vi "XYZ stage control.vi"() -> ()   [LabVIEW 2020]
panel:
  in  "Z down step size":dbl=100.0
  in  "Y down step size":dbl=100.0
  in  "X down step size":dbl=100.0
  out "X Position":dbl=-10.99177734375
  in  "X Step Size(um)":dbl=100.0
  in  "Right":bool
  in  "Left":bool
  out "Y Position":dbl=3.8870703125000023
  in  "Focus Down X":bool
  in  "Y Step Size(um)":dbl=100.0
  in  "Focus Up X":bool caption="Focus Up"
  in  "Focus Down":bool
  out "Z Position":dbl=6.860690000000502
  in  "Focus Up":bool
  in  "Z step size (um)":dbl=100.0
  in  "Close Communication":bool
  out "Error out":errorcluster
  out "Connected":bool=TRUE
  out "GetFirmwareVersion 2":string="3.03\r"
  in  "SPIIPLUSCOM660Lib.IAsyncChannel":refnum<k7>
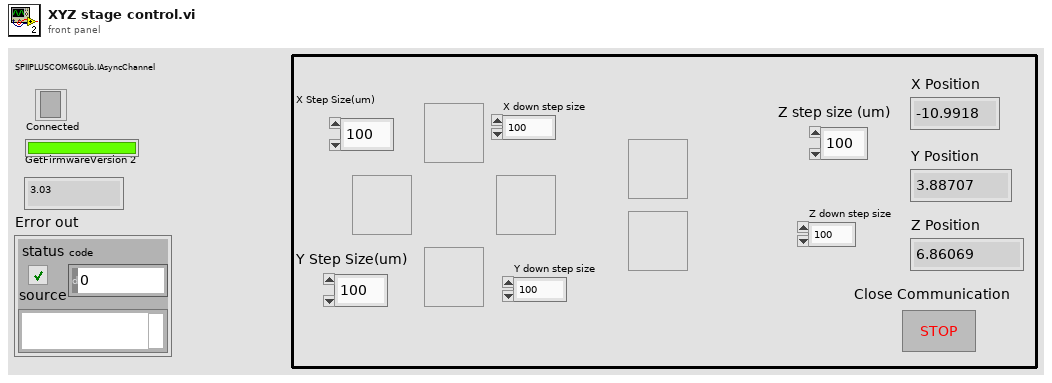
[diagram p1: front panel]
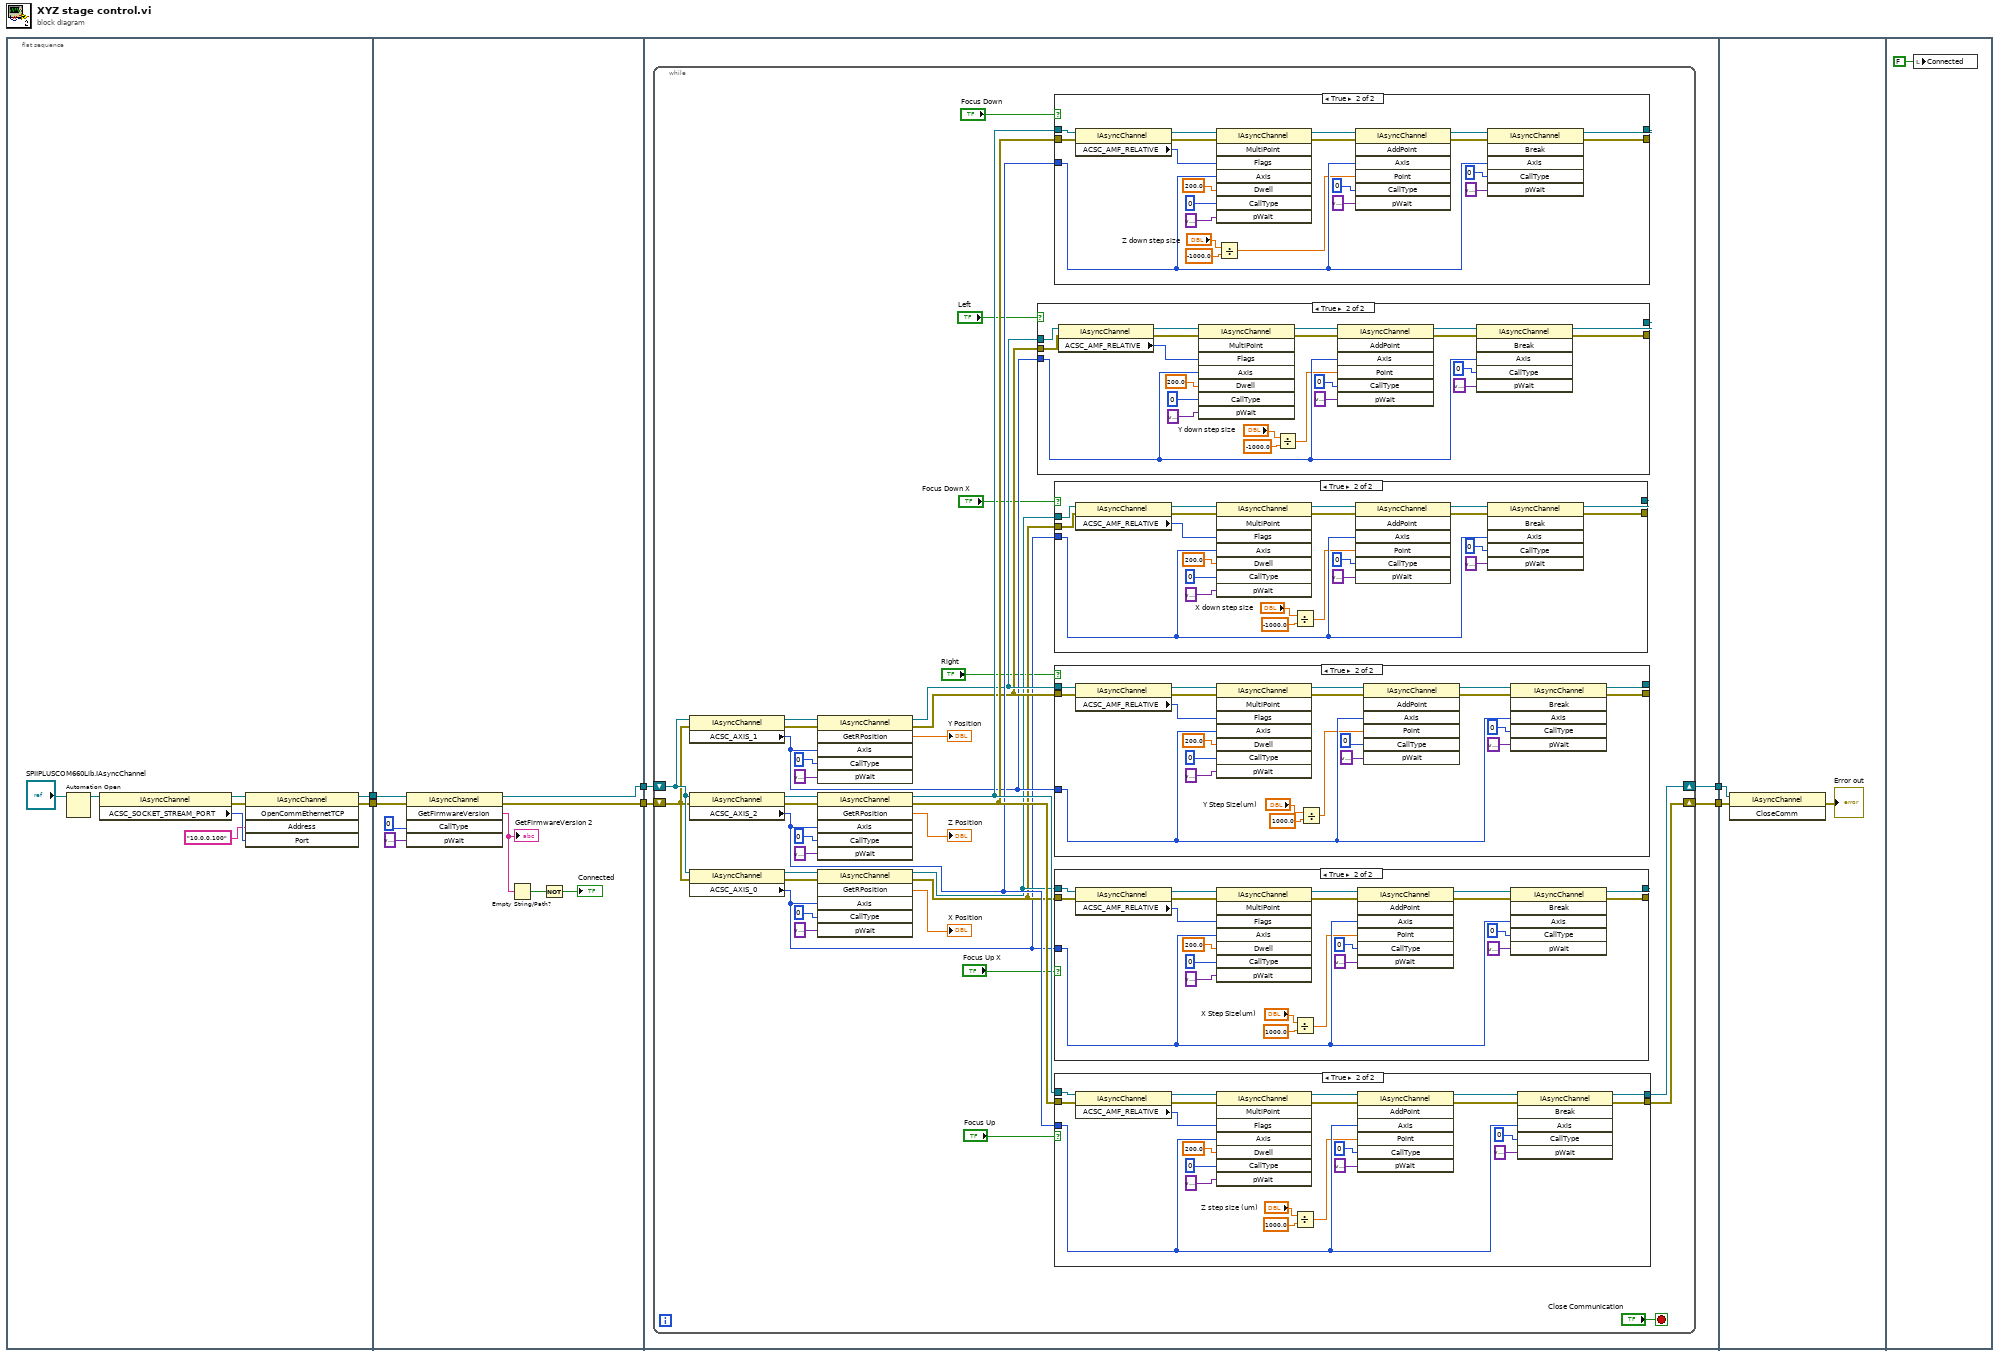
[diagram p0: block diagram]
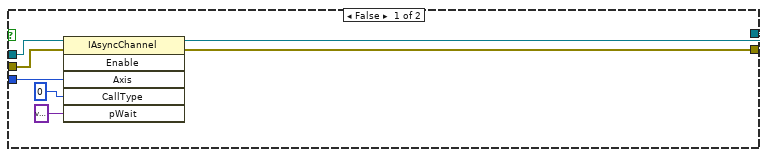
[diagram p2: hidden frame]
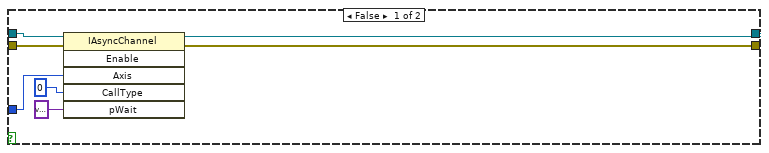
[diagram p3: hidden frame]
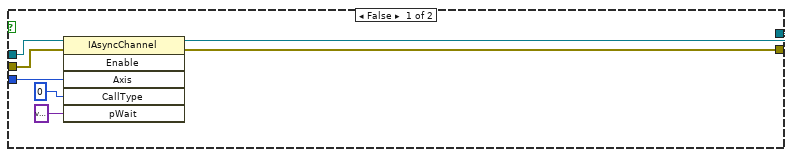
[diagram p4: hidden frame]
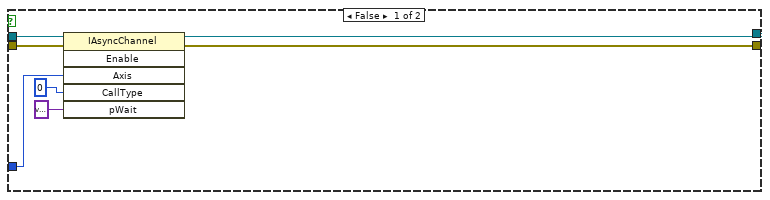
[diagram p5: hidden frame]
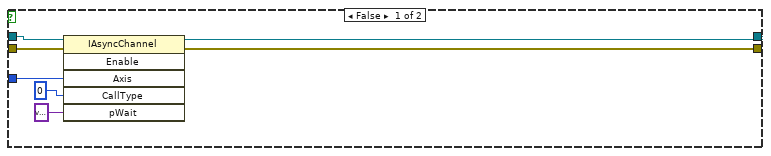
[diagram p6: hidden frame]
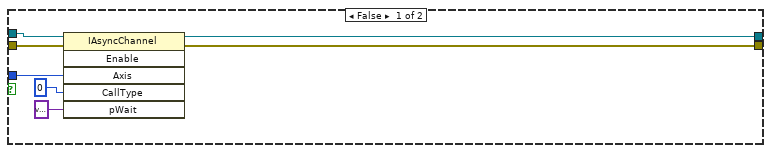
[diagram p7: hidden frame]
diagram:
  n1 = flat-sequence {
    tunnel: [w9] -> w6
    tunnel: [w8] -> w5
    tunnel: w6 -> [w19]
    tunnel: w5 -> [w18]
    tunnel: [w16] -> w4
    tunnel: [w15] -> w3
    tunnel: w4 -> [w24]
    tunnel: w3 -> [w27]
    tunnel: [w26] -> w2
    tunnel: [w25] -> w1
    tunnel: w2 -> [w238]
    tunnel: w1 -> [w237]
    frame #0 {
      n2 = Automation Open(Automation Refnum="SPIIPLUSCOM660Lib.IAsyncChannel") -> (Automation Refnum=w14:refnum<k7>)  [unwired: 3 in, 1 out]
      n3 = property class="IAsyncChannel"(reference=w14) -> (reference out=w13:refnum<k7>, error out=w7:errorcluster, "ACSC_SOCKET_STREAM_PORT"=w11:i32)  [unwired: 1 in]
      n4 = invoke class="IAsyncChannel" method="OpenCommEthernetTCP"(reference=w13, error in=w7, "Address"="10.0.0.100", "Port"=w11) -> (reference out=w9:refnum<k7>, error out=w8:errorcluster)  [unwired: 1 in, 3 out]
    }
    frame #1 {
      n5 = invoke class="IAsyncChannel" method="GetFirmwareVersion"(reference=w19, error in=w18, "CallType"=u64 0, "pWait"=variant) -> (reference out=w16:refnum<k7>, error out=w15:errorcluster, "GetFirmwareVersion"=w21:string)  [unwired: 1 in, 2 out]
      "GetFirmwareVersion 2" <- w21
      n6 = Empty String/Path?(string/path=w21) -> (empty?=w20:bool)
      n7 = Not(x=w20) -> (.not. x?=→"Connected":bool)
    }
    frame #2 {
      n8 = while {
        shift-right: [w62] -> w26
        shift-left: w24 -> [w41]
        shift-right: [w61] -> w25
        shift-left: w27 -> [w40]
        stop <- "Close Communication" stop-if-true
        n9 = property class="IAsyncChannel"(reference=w41, error in=w40) -> (reference out=w49:refnum<k7>, error out=w48:errorcluster, "ACSC_AXIS_1"=w45:i32)
        n10 = property class="IAsyncChannel"(reference=w41, error in=w40) -> (reference out=w58:refnum<k7>, error out=w57:errorcluster, "ACSC_AXIS_2"=w50:i32)
        n11 = property class="IAsyncChannel"(reference=w41, error in=w40) -> (reference out=w39:refnum<k7>, error out=w38:errorcluster, "ACSC_AXIS_0"=w34:i32)
        n12 = invoke class="IAsyncChannel" method="GetRPosition"(reference=w49, error in=w48, "Axis"=w45, "CallType"=u64 0, "pWait"=variant) -> (reference out=w47:refnum<k7>, error out=w46:errorcluster, "GetRPosition"=→"Y Position":dbl)  [unwired: 1 in, 3 out]
        n13 = invoke class="IAsyncChannel" method="GetRPosition"(reference=w58, error in=w57, "Axis"=w50, "CallType"=u64 0, "pWait"=variant) -> (reference out=w52:refnum<k7>, error out=w51:errorcluster, "GetRPosition"=→"Z Position":dbl)  [unwired: 1 in, 3 out]
        n14 = invoke class="IAsyncChannel" method="GetRPosition"(reference=w39, error in=w38, "Axis"=w34, "CallType"=u64 0, "pWait"=variant) -> (reference out=w36:refnum<k7>, error out=w35:errorcluster, "GetRPosition"=→"X Position":dbl)  [unwired: 1 in, 3 out]
        n15 = case shown="True" "Left" {
          tunnel: w47 -> [w127 w148]
          tunnel: w46 -> [w126 w149]
          tunnel: [w125 w132] -> _
          tunnel: [w124 w131] -> _
          tunnel: w45 -> [w123 w135]
          frame False {
            n16 = invoke class="IAsyncChannel" method="Enable"(reference=w127, error in=w126, "Axis"=w123, "CallType"=u64 0, "pWait"=variant) -> (reference out=w125:refnum<k7>, error out=w124:errorcluster)  [unwired: 1 in, 4 out]
          }
          frame True {
            n17 = property class="IAsyncChannel"(reference=w148, error in=w149) -> (reference out=w147:refnum<k7>, error out=w146:errorcluster, "ACSC_AMF_RELATIVE"=w143:i32)
            n18 = invoke class="IAsyncChannel" method="MultiPoint"(reference=w147, error in=w146, "Flags"=w143, "Axis"=w135, "Dwell"=200.0, "CallType"=u64 0, "pWait"=variant) -> (reference out=w142:refnum<k7>, error out=w141:errorcluster)  [unwired: 1 in, 6 out]
            n19 = Divide(x="Y down step size", y=-1000.0) -> (x/y=w129:dbl)
            n20 = invoke class="IAsyncChannel" method="AddPoint"(reference=w142, error in=w141, "Axis"=w135, "Point"=w129, "CallType"=u64 0, "pWait"=variant) -> (reference out=w137:refnum<k7>, error out=w136:errorcluster)  [unwired: 1 in, 5 out]
            n21 = invoke class="IAsyncChannel" method="Break"(reference=w137, error in=w136, "Axis"=w135, "CallType"=u64 0, "pWait"=variant) -> (reference out=w132:refnum<k7>, error out=w131:errorcluster)  [unwired: 1 in, 4 out]
          }
        }
        n22 = case shown="True" "Focus Down" {
          tunnel: w52 -> [w185 w206]
          tunnel: w51 -> [w184 w207]
          tunnel: [w183 w190] -> _
          tunnel: [w182 w189] -> _
          tunnel: w50 -> [w181 w193]
          frame False {
            n23 = invoke class="IAsyncChannel" method="Enable"(reference=w185, error in=w184, "Axis"=w181, "CallType"=u64 0, "pWait"=variant) -> (reference out=w183:refnum<k7>, error out=w182:errorcluster)  [unwired: 1 in, 4 out]
          }
          frame True {
            n24 = property class="IAsyncChannel"(reference=w206, error in=w207) -> (reference out=w205:refnum<k7>, error out=w204:errorcluster, "ACSC_AMF_RELATIVE"=w201:i32)
            n25 = invoke class="IAsyncChannel" method="MultiPoint"(reference=w205, error in=w204, "Flags"=w201, "Axis"=w193, "Dwell"=200.0, "CallType"=u64 0, "pWait"=variant) -> (reference out=w200:refnum<k7>, error out=w199:errorcluster)  [unwired: 1 in, 6 out]
            n26 = Divide(x="Z down step size", y=-1000.0) -> (x/y=w187:dbl)
            n27 = invoke class="IAsyncChannel" method="AddPoint"(reference=w200, error in=w199, "Axis"=w193, "Point"=w187, "CallType"=u64 0, "pWait"=variant) -> (reference out=w195:refnum<k7>, error out=w194:errorcluster)  [unwired: 1 in, 5 out]
            n28 = invoke class="IAsyncChannel" method="Break"(reference=w195, error in=w194, "Axis"=w193, "CallType"=u64 0, "pWait"=variant) -> (reference out=w190:refnum<k7>, error out=w189:errorcluster)  [unwired: 1 in, 4 out]
          }
        }
        n29 = case shown="True" "Focus Down X" {
          tunnel: w36 -> [w69 w90]
          tunnel: w35 -> [w68 w91]
          tunnel: [w67 w74] -> _
          tunnel: [w66 w73] -> _
          tunnel: w34 -> [w65 w77]
          frame False {
            n30 = invoke class="IAsyncChannel" method="Enable"(reference=w69, error in=w68, "Axis"=w65, "CallType"=u64 0, "pWait"=variant) -> (reference out=w67:refnum<k7>, error out=w66:errorcluster)  [unwired: 1 in, 4 out]
          }
          frame True {
            n31 = property class="IAsyncChannel"(reference=w90, error in=w91) -> (reference out=w89:refnum<k7>, error out=w88:errorcluster, "ACSC_AMF_RELATIVE"=w85:i32)
            n32 = invoke class="IAsyncChannel" method="MultiPoint"(reference=w89, error in=w88, "Flags"=w85, "Axis"=w77, "Dwell"=200.0, "CallType"=u64 0, "pWait"=variant) -> (reference out=w84:refnum<k7>, error out=w83:errorcluster)  [unwired: 1 in, 6 out]
            n33 = Divide(x="X down step size", y=-1000.0) -> (x/y=w71:dbl)
            n34 = invoke class="IAsyncChannel" method="AddPoint"(reference=w84, error in=w83, "Axis"=w77, "Point"=w71, "CallType"=u64 0, "pWait"=variant) -> (reference out=w79:refnum<k7>, error out=w78:errorcluster)  [unwired: 1 in, 5 out]
            n35 = invoke class="IAsyncChannel" method="Break"(reference=w79, error in=w78, "Axis"=w77, "CallType"=u64 0, "pWait"=variant) -> (reference out=w74:refnum<k7>, error out=w73:errorcluster)  [unwired: 1 in, 4 out]
          }
        }
        n36 = case shown="True" "Right" {
          tunnel: w47 -> [w156 w177]
          tunnel: w46 -> [w155 w178]
          tunnel: [w154 w161] -> _
          tunnel: [w153 w160] -> _
          tunnel: w45 -> [w152 w164]
          frame False {
            n37 = invoke class="IAsyncChannel" method="Enable"(reference=w156, error in=w155, "Axis"=w152, "CallType"=u64 0, "pWait"=variant) -> (reference out=w154:refnum<k7>, error out=w153:errorcluster)  [unwired: 1 in, 4 out]
          }
          frame True {
            n38 = property class="IAsyncChannel"(reference=w177, error in=w178) -> (reference out=w176:refnum<k7>, error out=w175:errorcluster, "ACSC_AMF_RELATIVE"=w172:i32)
            n39 = invoke class="IAsyncChannel" method="MultiPoint"(reference=w176, error in=w175, "Flags"=w172, "Axis"=w164, "Dwell"=200.0, "CallType"=u64 0, "pWait"=variant) -> (reference out=w171:refnum<k7>, error out=w170:errorcluster)  [unwired: 1 in, 6 out]
            n40 = Divide(x="Y Step Size(um)", y=1000.0) -> (x/y=w158:dbl)
            n41 = invoke class="IAsyncChannel" method="AddPoint"(reference=w171, error in=w170, "Axis"=w164, "Point"=w158, "CallType"=u64 0, "pWait"=variant) -> (reference out=w166:refnum<k7>, error out=w165:errorcluster)  [unwired: 1 in, 5 out]
            n42 = invoke class="IAsyncChannel" method="Break"(reference=w166, error in=w165, "Axis"=w164, "CallType"=u64 0, "pWait"=variant) -> (reference out=w161:refnum<k7>, error out=w160:errorcluster)  [unwired: 1 in, 4 out]
          }
        }
        n43 = case shown="True" "Focus Up X" {
          tunnel: w36 -> [w98 w119]
          tunnel: w35 -> [w97 w120]
          tunnel: [w96 w103] -> _
          tunnel: [w95 w102] -> _
          tunnel: w34 -> [w94 w106]
          frame False {
            n44 = invoke class="IAsyncChannel" method="Enable"(reference=w98, error in=w97, "Axis"=w94, "CallType"=u64 0, "pWait"=variant) -> (reference out=w96:refnum<k7>, error out=w95:errorcluster)  [unwired: 1 in, 4 out]
          }
          frame True {
            n45 = property class="IAsyncChannel"(reference=w119, error in=w120) -> (reference out=w118:refnum<k7>, error out=w117:errorcluster, "ACSC_AMF_RELATIVE"=w114:i32)
            n46 = invoke class="IAsyncChannel" method="MultiPoint"(reference=w118, error in=w117, "Flags"=w114, "Axis"=w106, "Dwell"=200.0, "CallType"=u64 0, "pWait"=variant) -> (reference out=w113:refnum<k7>, error out=w112:errorcluster)  [unwired: 1 in, 6 out]
            n47 = Divide(x="X Step Size(um)", y=1000.0) -> (x/y=w100:dbl)
            n48 = invoke class="IAsyncChannel" method="AddPoint"(reference=w113, error in=w112, "Axis"=w106, "Point"=w100, "CallType"=u64 0, "pWait"=variant) -> (reference out=w108:refnum<k7>, error out=w107:errorcluster)  [unwired: 1 in, 5 out]
            n49 = invoke class="IAsyncChannel" method="Break"(reference=w108, error in=w107, "Axis"=w106, "CallType"=u64 0, "pWait"=variant) -> (reference out=w103:refnum<k7>, error out=w102:errorcluster)  [unwired: 1 in, 4 out]
          }
        }
        n50 = case shown="True" "Focus Up" {
          tunnel: w52 -> [w214 w235]
          tunnel: w51 -> [w213 w236]
          tunnel: [w212 w219] -> w62
          tunnel: [w211 w218] -> w61
          tunnel: w50 -> [w210 w222]
          frame False {
            n51 = invoke class="IAsyncChannel" method="Enable"(reference=w214, error in=w213, "Axis"=w210, "CallType"=u64 0, "pWait"=variant) -> (reference out=w212:refnum<k7>, error out=w211:errorcluster)  [unwired: 1 in, 4 out]
          }
          frame True {
            n52 = property class="IAsyncChannel"(reference=w235, error in=w236) -> (reference out=w234:refnum<k7>, error out=w233:errorcluster, "ACSC_AMF_RELATIVE"=w230:i32)
            n53 = invoke class="IAsyncChannel" method="MultiPoint"(reference=w234, error in=w233, "Flags"=w230, "Axis"=w222, "Dwell"=200.0, "CallType"=u64 0, "pWait"=variant) -> (reference out=w229:refnum<k7>, error out=w228:errorcluster)  [unwired: 1 in, 6 out]
            n54 = Divide(x="Z step size (um)", y=1000.0) -> (x/y=w216:dbl)
            n55 = invoke class="IAsyncChannel" method="AddPoint"(reference=w229, error in=w228, "Axis"=w222, "Point"=w216, "CallType"=u64 0, "pWait"=variant) -> (reference out=w224:refnum<k7>, error out=w223:errorcluster)  [unwired: 1 in, 5 out]
            n56 = invoke class="IAsyncChannel" method="Break"(reference=w224, error in=w223, "Axis"=w222, "CallType"=u64 0, "pWait"=variant) -> (reference out=w219:refnum<k7>, error out=w218:errorcluster)  [unwired: 1 in, 4 out]
          }
        }
      }
    }
    frame #3 {
      n57 = invoke class="IAsyncChannel" method="CloseComm"(reference=w238, error in=w237) -> (error out=→"Error out":errorcluster)  [unwired: 1 in, 2 out]
    }
    frame #4 {
      n58 = local write "Connected"(FALSE ("Connected")) -> ()
    }
  }
